vi "GetIpAddressFromConectionInfo.vi"(8 "Error in":errorcluster, 11 "ConnectionInfo":refnum<k24>) -> (0 "Error out":errorcluster, 2 "Port":i32, 3 "IpAddress":string)   [LabVIEW 2016]
doc: "Get the IP address and the port of a connection info."
uses:
  C:/Users/CL/Desktop/ZcDAQprj0811/ZcDAQprj/Modules/DAQ-Device/Hardware Drivers/QX/HBM LabVIEW Driver/DLLs/Hbm.Api.Common.dll
  DLLs/Hbm.Api.Common.dll
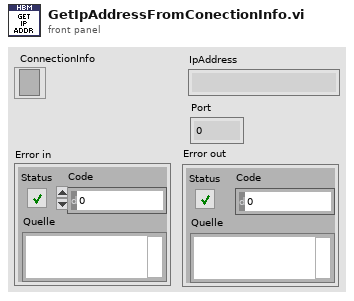
[diagram p1: front panel]
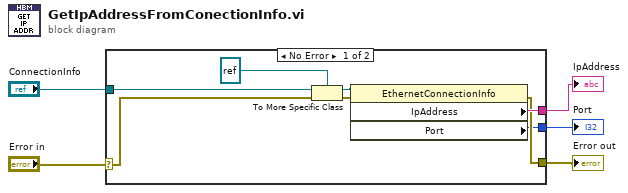
[diagram p0: block diagram]
diagram:
  n1 = case shown="No Error" "Error in" {
    selector: "Error in" -> [w6 w14]
    tunnel: [w13 _] -> w5
    tunnel: [w12 w14] -> w4
    tunnel: [w11 _] -> w3
    tunnel: "ConnectionInfo" -> [w8 _]
    frame No Error {
      n2 = To More Specific Class(target class=refnum<k24> refnum (".NET (Referenz)"), reference=w8, error in=w6) -> (specific class reference=w9:refnum<k24>, error out=w10:errorcluster)
      n3 = property on="Eigenschaftsknoten" class="EthernetConnectionInfo"(reference=w9, error in=w10) -> (error out=w12:errorcluster, "IpAddress"=w13:string, "Port"=w11:i32)  [unwired: 1 out]
    }
    frame Error {
    }
  }
  "IpAddress" <- w5
  "Error out" <- w4
  "Port" <- w3
